vi "Speech Recognizer Initialize.vi"(8 "Error In":errorcluster, 9 "String[] phrases":string[](array[string]), 10 "Score":refnum<vi>, 11 "Text":refnum<vi>) -> (0 "error out":errorcluster, 2 "Event Callback":refnum<k27>, 3 "reference":refnum<k24>)   [LabVIEW 2013]
uses:
  System.Speech
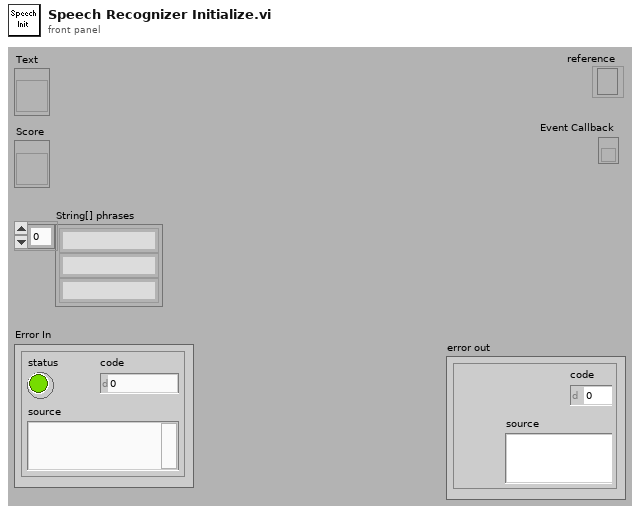
[diagram p1: front panel]
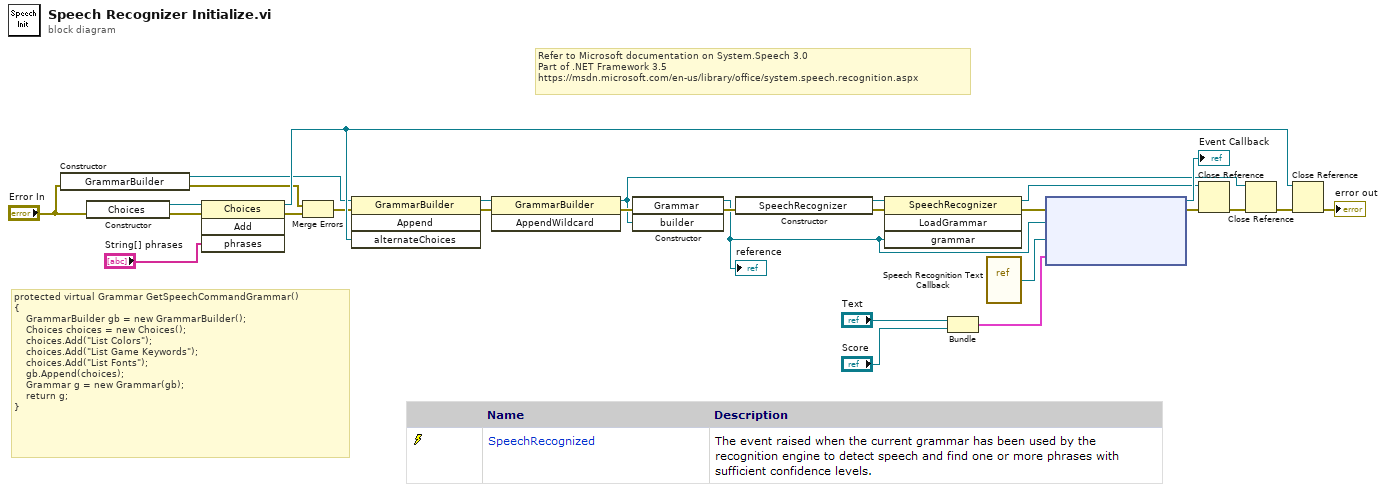
[diagram p0: block diagram]
diagram:
  # "protected virtual Grammar GetSpeechCommandGrammar()\n{\n    GrammarBuilder gb = new GrammarBuilder();\n    Choices choices = new Choices();\n    choices.Add(\"List Colors\");\n    choices.Add(\"List Game Keywords\");\n    choices.Add(\"List Fonts\");\n    gb.Append(choices);\n    Grammar g = new Grammar(gb);\n    return g;\n}"
  # "Refer to Microsoft documentation on System.Speech 3.0\nPart of .NET Framework 3.5\nhttps://msdn.microsoft.com/en-us/library/office/system.speech.recognition.aspx"
  n1 = constructor class="GrammarBuilder"(error in="Error In") -> (reference out=w5:refnum<k24>, error out=w10:errorcluster)  [unwired: 2 in, 1 out]
  n2 = constructor class="Choices"(error in="Error In") -> (reference out=w7:refnum<k24>, error out=w12:errorcluster)  [unwired: 2 in, 1 out]
  n3 = invoke class="Choices" method="Add"(reference=w7, error in=w12, "phrases"="String[] phrases") -> (reference out=w16:refnum<k24>, error out=w9:errorcluster)  [unwired: 1 in, 2 out]
  n4 = Merge Errors(w10, w9) -> (w11:errorcluster)
  n5 = invoke class="GrammarBuilder" method="Append"(reference=w5, error in=w11, "alternateChoices"=w16) -> (reference out=w8:refnum<k24>, error out=w6:errorcluster)  [unwired: 1 in, 2 out]
  n6 = invoke class="GrammarBuilder" method="AppendWildcard"(reference=w8, error in=w6) -> (reference out=w17:refnum<k24>, error out=w18:errorcluster)  [unwired: 1 in, 1 out]
  n7 = constructor class="Grammar"(error in=w18, "builder"=w17) -> (reference out=w3:refnum<k24>, error out=w15:errorcluster)  [unwired: 2 in, 2 out]
  "reference" <- w3
  n8 = constructor class="SpeechRecognizer"(error in=w15) -> (reference out=w24:refnum<k24>, error out=w25:errorcluster)  [unwired: 2 in, 1 out]
  n9 = invoke class="SpeechRecognizer" method="LoadGrammar"(reference=w24, error in=w25, "grammar"=w3) -> (reference out=w14:refnum<k24>, error out=w23:errorcluster)  [unwired: 1 in, 2 out]
  n10 = Bundle("Text"="Text", "Score"="Score") -> (w1:cluster{"Text":refnum<vi>, "Score":refnum<vi>})  [unwired: 1 out]
  n11 = vi-ref "Speech Recognition Text Callback.vi"() -> (w2:refnum<vi>)
  n12 = node(w23, w3, w2, w1) -> (→"Event Callback":refnum<k27>, w22:errorcluster)  [unwired: 1 in]
  n13 = Close Reference(reference=w14, error in (no error)=w22) -> (error out=w28:errorcluster)
  n14 = Close Reference(reference=w17, error in (no error)=w28) -> (error out=w27:errorcluster)
  n15 = Close Reference(reference=w16, error in (no error)=w27) -> (error out=→"error out":errorcluster)
